vi "Add Or Replace Img Array.vi"(8 "Img":u8[][](array[numeric]), 9 "Index":i32, 11 "Img Array In":u8[][][](array[numeric])) -> (3 "Img Array Out":u8[][][](array[numeric]))   [LabVIEW 2013]
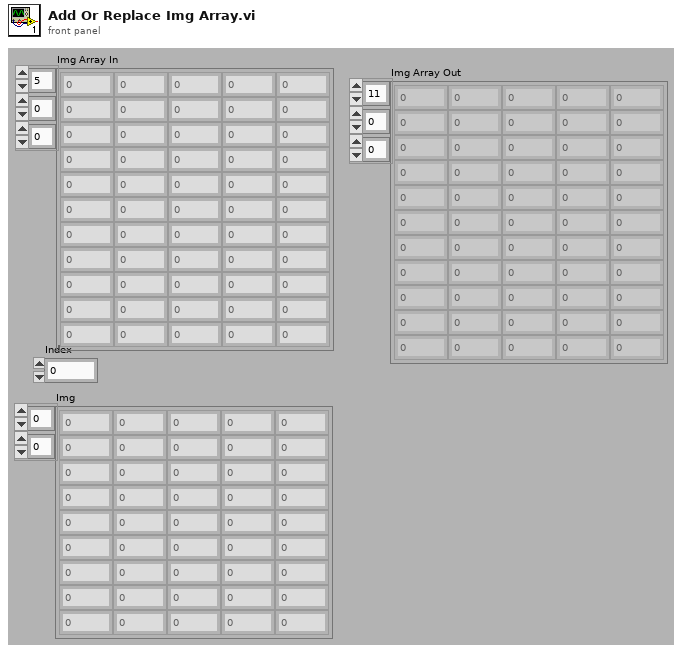
[diagram p1: front panel]
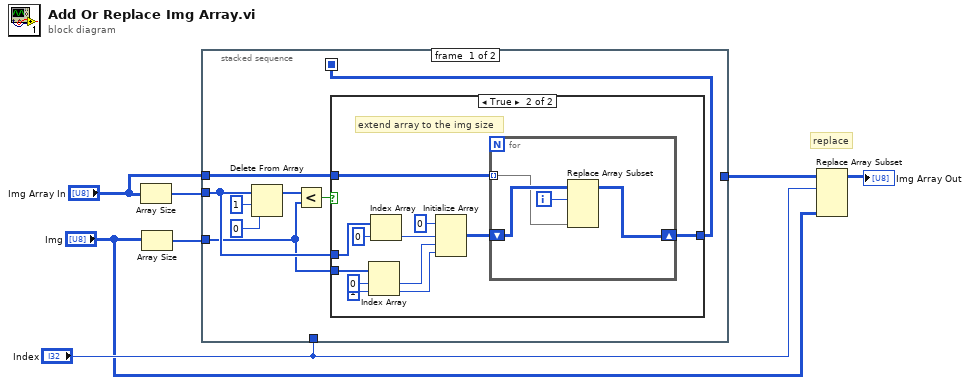
[diagram p0: block diagram]
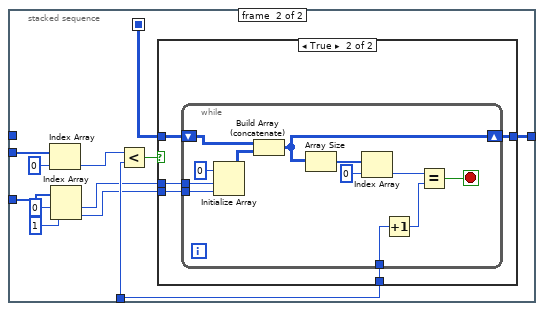
[diagram p3: hidden frame]
diagram:
  # "replace"
  n1 = Array Size(array="Img Array In") -> (size(s)=w2:i32[])
  n2 = Array Size(array="Img") -> (size(s)=w1:i32[])
  n3 = stacked-sequence {
    seq-local: [w10 _] -> [_ w33]
    tunnel: [_ w44] -> w7
    tunnel: "Index" -> [_ w43]
    tunnel: "Img Array In" -> [w11 _]
    tunnel: w2 -> [w9 w35]
    tunnel: w1 -> [w8 w34]
    frame #0 {
      n4 = Delete From Array(array=w9, length=1, index=0) -> (array with subset deleted=w13:i32[])  [unwired: 1 out]
      n5 = Less?(x=w13, y=w8) -> (x < y?=w12:bool)
      n6 = case shown="True" w12 {
        tunnel: w11 -> [w16 w26]
        tunnel: [w16 w24] -> w10
        tunnel: w9 -> [_ w23]
        tunnel: w8 -> [_ w21]
        frame False {
        }
        frame True {
          # "extend array to the img size"
          n7 = Index Array(array=w21, index #1=0 ("index"), index #2=1 ("index")) -> (element #1=w18:i32, element #2=w17:i32)
          n8 = Index Array(array=w23, index=0) -> (element=w27:i32)
          n9 = Initialize Array(u8 0 ("element"), w27, w18, w17) -> (w25:u8[][][])
          n10 = for {
            tunnel: w26 -> [w31] mode=indexing
            shift-right: [w29] -> w24
            shift-left: w25 -> [w32]
            i -> [w30]
            n11 = Replace Array Subset(array=w32, new element=w31, index (dim 0)=w30) -> (w29:u8[][][])  [unwired: 2 in]
          }
        }
      }
    }
    frame #1 {
      n12 = Index Array(array=w35, index=0) -> (element=w41:i32)
      n13 = Index Array(array=w34, index #1=0 ("index"), index #2=1 ("index")) -> (element #1=w38:i32, element #2=w37:i32)
      n14 = Less?(x=w41, y=w43) -> (x < y?=w40:bool)
      n15 = case shown="True" w40 {
        tunnel: [w45 w50] -> w44
        tunnel: w43 -> [_ w49]
        tunnel: w38 -> [_ w48]
        tunnel: w37 -> [_ w47]
        tunnel: w33 -> [w45 w46]
        frame False {
        }
        frame True {
          n16 = while {
            shift-right: [w62] -> w50
            shift-left: w46 -> [w51]
            tunnel: w49 -> [w61]
            tunnel: w48 -> [w53]
            tunnel: w47 -> [w52]
            stop <- w60 stop-if-true
            n17 = Initialize Array(u8 0, w53, w52) -> (w54:u8[][])
            n18 = Build Array (concatenate)(w51, w54) -> (w62:u8[][][])
            n19 = Array Size(array=w62) -> (size(s)=w57:i32[])
            n20 = Index Array(array=w57, index=0) -> (element=w56:i32)
            n21 = Increment(x=w61) -> (x+1=w59:i32)
            n22 = Equal?(x=w56, y=w59) -> (x = y?=w60:bool)
          }
        }
      }
    }
  }
  n23 = Replace Array Subset(array=w7, new element="Img", index (dim 0)="Index") -> (→"Img Array Out":u8[][][])  [unwired: 2 in]
